vi "Warning_Valori_inferiori_soglia.vi"(8 "error in (no error)":errorcluster, 9 "Enable":bool=TRUE, 10 "Message":string="WARNING: Valori inferiori rispetto alle soglie impostate ") -> (0 "error out":errorcluster, 2 "Avanti":bool)   [LabVIEW 2023]
doc: "Displays a standard dialog box that contains an alert or a message for users.\n--------------------\n\nThis Express VI is configured as follows:\n\nMessage: WARNING: Valori inferiori rispetto alle soglie impostate"
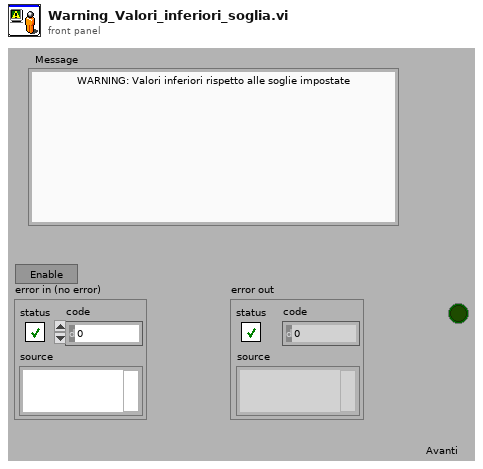
[diagram p1: front panel]
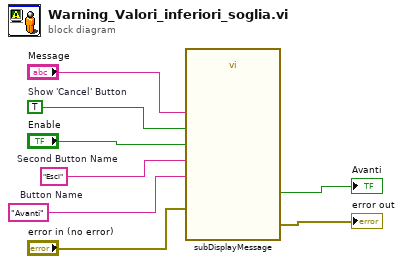
[diagram p0: block diagram]
diagram:
  w3 = "Avanti"  # Button Name
  w4 = "Esci"  # Second Button Name
  w6 = TRUE  # Show 'Cancel' Button
  n1 = call <vilib>:"subDisplayMessage.vi"("Second Button Name"=w4, "Button Name"=w3, "error in (no error)"="error in (no error)", "Enable Message"="Enable", "Show 'Cancel' Button"=w6, "Message to Display"="Message") -> ("error out"=→"error out":errorcluster, "OK?"=→"Avanti":bool)  [unwired: 4 in]
